vi "Default INITextManager Object.vi"(11 "CfgManager.Text.INI in":refnum<class "ConfigManager.Text.INI.lvclass">) -> (3 "CfgManager.Text.INI out":refnum<class "ConfigManager.Text.INI.lvclass">)   [LabVIEW 2013, in "CfgManager.Text.lvlib" / "ConfigManager.Text.INI.lvclass"]
uses:
  ConfigManager.Text.INI.lvclass
  <vilib>/LabVIEW Open Source Project/Unicity/Delimiter/Delimiters List.ctl
  <vilib>/LabVIEW Open Source Project/Serializer/Serializer.INI/Serializer.PlainText.INI.lvclass
  Manager.Text/ConfigManager.Text.lvclass/ConfigManager.Text.ctl
  Manager/ConfigManager.lvclass/ConfigManager.ctl
  <vilib>/LabVIEW Open Source Project/Unicity/Delimiter/Delimiter.lvclass
  Manager/ConfigManager.lvclass
  Manager.Text/ConfigManager.Text.lvclass
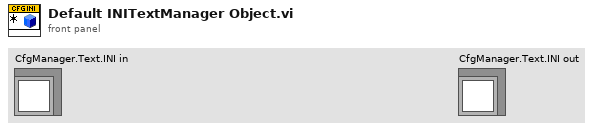
[diagram p1: front panel]
types:
  T1 = typedef "Delimiter.lvclass/Delimiters List.ctl" = enum16{"Default", "dot (.)", "colon (:)", "double-colon (::)", "semi-colon (;)", "underscore (_)", "double underscore (__)", "dash (-)", "double dash (--)", "backslash (\\)", "vertical bar (|)", "forward slash (/)", "chevron (>)", "double-chevron (>>)", "arrow (->)", "comma (,)", "arobas (@)", "ampersand (&)", "other"}
  T2 = typedef "CfgManager.Text.lvlib/ConfigManager.Text.lvclass/Configuration -- Cluster.ctl" = cluster{"FileHeader":refnum<class "FileHeader.lvclass">, "FileSignature":refnum<class "FileSignature.lvclass">, "Section Delimiter":refnum<class "Delimiter.lvclass">, "Key-Value Separator":refnum<class "Delimiter.lvclass">}
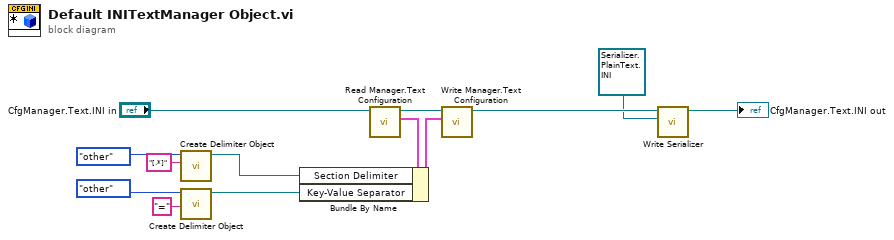
[diagram p0: block diagram]
diagram:
  n1 = call <vilib>:"Create Delimiter Object.vi"("Other"="[.*]", "Delimiter"=Delimiters_List."other") -> ("Delimiter"=w10:refnum<class "Delimiter.lvclass">)  [unwired: 9 in]
  n2 = call <vilib>:"Create Delimiter Object.vi"("Other"="=", "Delimiter"=Delimiters_List."other") -> ("Delimiter"=w9:refnum<class "Delimiter.lvclass">)  [unwired: 9 in]
  n3 = call "Read Manager.Text Configuration.vi"("ConfigManager.Text in"="CfgManager.Text.INI in") -> ("Manager.Text Configuration"=w8:T2, "ConfigManager.Text out"=w4:refnum<class "ConfigManager.Text.INI.lvclass">)  [unwired: 9 in]
  n4 = Bundle By Name(cluster=w8, "Section Delimiter"=w10, "Key-Value Separator"=w9) -> (w3:T2)
  n5 = call "Write Manager.Text Configuration.vi"("Manager.Text Configuration"=w3, "ConfigManager.Text in"=w4) -> ("ConfigManager.Text out"=w5:refnum<class "ConfigManager.Text.INI.lvclass">)  [unwired: 9 in]
  n6 = call "Write Serializer.vi"("Serializer"=refnum<class "Serializer.PlainText.INI.lvclass"> refnum ("Serializer.PlainText.INI"), "ConfigManager in"=w5) -> ("ConfigManager out"=→"CfgManager.Text.INI out":refnum<class "ConfigManager.Text.INI.lvclass">)  [unwired: 9 in]
